vi "LimitFlagActionSoftLinearizedT.vi"(4 "Soft":bool, 5 "Axis limit flag":bool, 6 "Old Control":dbl, 7 "Global limit flag active":dbl, 8 "Stop motors global":bool, 9 "Stop motor local":bool, 10 "Axis control signal":dbl) -> (0 "Slider control":dbl, 1 "PWM Brake":u32, 2 "PWM Direction":u32, 3 "PWM width":u32)   [LabVIEW 2009]
uses:
  <vilib>/imath/engines/lvmath2/RunTimeEngine/ErrorHandling/NIMS_Finalize Error.vi
  <vilib>/imath/engines/lvmath2/RunTimeEngine/Parser/MC_Version.vi
  <vilib>/imath/engines/lvmath/Functions/Error Handling/MergeErrorsWrapper.vi
  <vilib>/imath/engines/lvmath2/RunTimeEngine/VariableToken/NIMS_VariableToken_CondDefined.vi
  <instcachedir>/0/NIMS_VariableToken_CondDefined_8A7BE13368864D8DBC6F49EC23B20D8F.lvgen/NIMS_VariableToken_CondDefined_8A7BE13368864D8DBC6F49EC23B20D8F_000.vi
  <instcachedir>/0/NIMS_VariableToken_CondDefined_8A7BE13368864D8DBC6F49EC23B20D8F.lvgen/NIMS_VariableToken_CondDefined_8A7BE13368864D8DBC6F49EC23B20D8F_001.vi
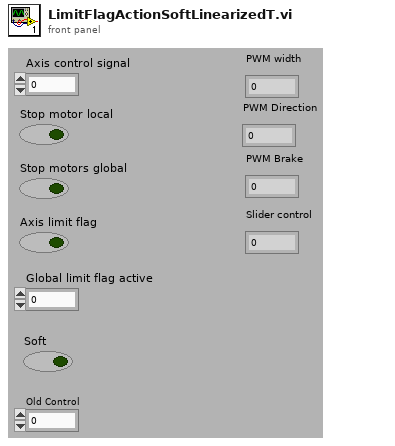
[diagram p1: front panel]
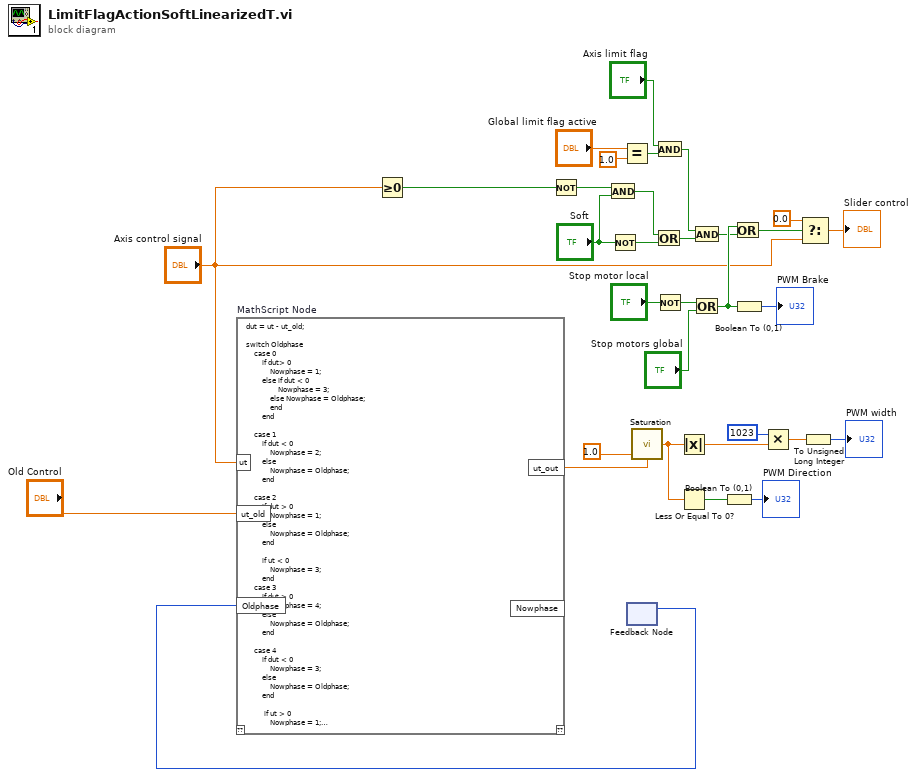
[diagram p0: block diagram]
diagram:
  n1 = Greater Or Equal To 0?(x="Axis control signal") -> (x >= 0?=w13:bool)
  n2 = Not(x=w13) -> (.not. x?=w12:bool)
  n3 = And(x=w12, y="Soft") -> (x .and. y?=w11:bool)
  n4 = Not(x="Soft") -> (.not. x?=w10:bool)
  n5 = Equal?(x="Global limit flag active", y=1.0) -> (x = y?=w31:bool)
  n6 = feedback #1() -> (w1:i32)  [unwired: 1 in]
  n7 = mathscript code="dut = ut - ut_old;\n\nswitch Oldphase\n    case 0\n        if dut> 0\n            Nowphase = 1;\n        else if dut < 0\n                Nowphase = 3;\n            else Nowphase = Oldphase;\n            end\n        end\n        \n    case 1\n        if dut < 0\n            Nowphase = 2;\n        else\n            Nowphase = Oldphase;\n        end\n        \n    case 2\n        if dut > 0\n            Nowphase = 1;\n        else\n            Nowphase = Oldphase;\n        end\n        \n        if ut < 0\n            Nowphase = 3;\n        end\n    case 3\n        if dut > 0\n            Nowphase = 4;\n        else\n            Nowphase = Oldphase;\n        end\n        \n    case 4\n        if dut < 0\n            Nowphase = 3;\n        else\n            Nowphase = Oldphase;\n        end\n\n         if ut > 0\n            Nowphase = 1;\n        end\n\nend\n\nif ut == 0\n    Nowphase = 0;\nend\n\n% Compensate input in different phases\nswitch Nowphase\n    case 0\n        ut_out = 0;\n    case 1\n        ut_out = 0.725*ut + 0.212;\n    case 2\n        ut_out = ut + 0.155;\n    case 3\n        ut_out = 0.7304*ut - 0.2288;\n    case 4\n        ut_out = ut - 0.1;\nend\n%\n% if ut_old*ut<=0\n%ut_out=-5*ut\n%end\n\n% Saturation\nif ut_out > 1\n    ut_out = 1;\nend\nif ut_out < -1\n    ut_out = -1;\nend"("ut"="Axis control signal", "ut_old"="Old Control", "Oldphase"=w1) -> ("ut_out"=w6:dbl, "Nowphase"=w2:i32)  [unwired: 1 in, 1 out]
  n8 = call "Saturation.vi"("Limit"=1.0, "Input"=w6) -> ("Output"=w4:dbl)
  n9 = Or(x=w11, y=w10) -> (x .or. y?=w8:bool)
  n10 = And(x="Axis limit flag", y=w31) -> (x .and. y?=w14:bool)
  n11 = Not(x="Stop motor local") -> (.not. x?=w33:bool)
  n12 = Absolute Value(x=w4) -> (abs(x)=w24:dbl)
  n13 = Less Or Equal To 0?(x=w4) -> (x <= 0?=w21:bool)
  n14 = And(x=w14, y=w8) -> (x .and. y?=w15:bool)
  n15 = Or(x=w33, y="Stop motors global") -> (x .or. y?=w17:bool)
  n16 = Boolean To (0,1)(Boolean=w21) -> (0, 1=→"PWM Direction":i16)
  n17 = Or(x=w17, y=w15) -> (x .or. y?=w18:bool)
  n18 = Boolean To (0,1)(Boolean=w17) -> (0, 1=→"PWM Brake":i16)
  n19 = Multiply(x=1023, y=w24) -> (x*y=w22:dbl)
  n20 = Select(t=0.0, s=w18, f="Axis control signal") -> (s? t:f=→"Slider control":dbl)
  n21 = To Unsigned Long Integer(number=w22) -> (unsigned 32bit integer=→"PWM width":u32)
